vi "Write System State Ref.vi"(8 "error in (no error)":errorcluster, 10 "System Status Ref":refnum<vi>, 11 "System Actor in":refnum<class "System Actor.lvclass">) -> (0 "error out":errorcluster, 3 "System Actor out":refnum<class "System Actor.lvclass">)   [LabVIEW 2014, in "Robot Actor Framework.lvlib" / "System Actor.lvlib" / "System Actor.lvclass"]
uses:
  System Actor.lvclass
  System State.ctl
  Command Actor/Command Actor Class/Command State.ctl
  Command Actor/Command Actor Class/Command States.ctl
  Command Processor Actor/Command Processor Actor Class/Command Processor State.ctl
  Command Processor Actor/Command Processor Actor Class/Command Processor States.ctl
  System Actor.lvclass/System Actor.ctl
  Command Actor/Command Actor Class/Command Actor.lvclass
  Command Processor Actor/Command Processor Actor Class/Command Processor Actor.lvclass
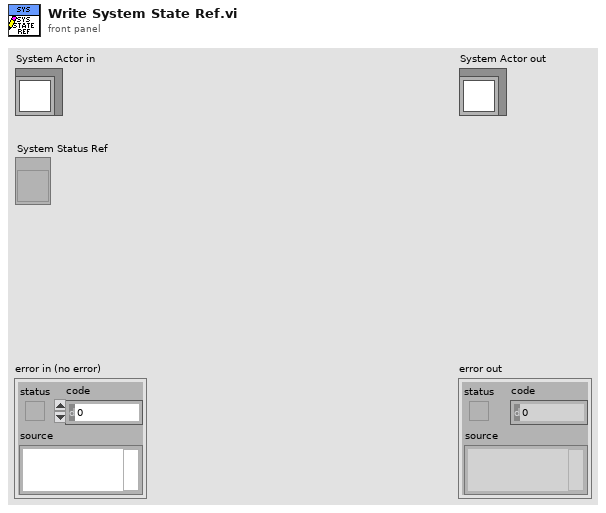
[diagram p1: front panel]
types:
  T1 = typedef "Robot Actor Framework.lvlib/System Actor.lvlib/System Actor.lvclass/System State.ctl" = cluster{"Instance Name":string, "Current Command Status":T2, "System Start Time":timestamp, "Next Command ID":dbl, "Command Processor Status":T4}
  T2 = typedef "Robot Actor Framework.lvlib/Command Actor.lvlib/Command Actor.lvclass/Command State.ctl" = cluster{"Command Name":string, "Command Start Time":timestamp, "Command End Time":timestamp, "Is Command Finished?":bool, "Command ID":u32, "Command State":T3, "Command State Time":timestamp}
  T3 = typedef "Robot Actor Framework.lvlib/Command Actor.lvlib/Command Actor.lvclass/Command States.ctl" = enum16{"Unknown", "Started", "Stopped", "Finished"}
  T4 = typedef "Robot Actor Framework.lvlib/Command Processor Actor.lvlib/Command Processor Actor.lvclass/Command Processor State.ctl" = cluster{"Current State":T5, "Last State Update":timestamp, "Queued Commands":u32, "Current Command Status":T2, "Previous State":T5, "Current State Entry":timestamp, "Transitioning State":bool, "Commands Behind":dbl, "Last Command Queue Time":timestamp}
  T5 = typedef "Robot Actor Framework.lvlib/Command Processor Actor.lvlib/Command Processor Actor.lvclass/Command Processor States.ctl" = enum16{"Unknown", "No Command", "Running Command", "Starting Command", "Stopping Command", "Finishing Command"}
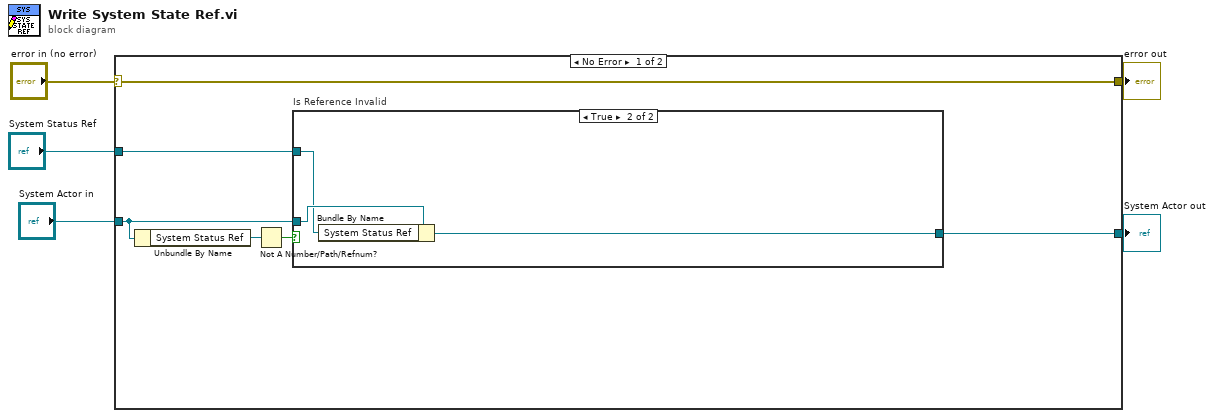
[diagram p0: block diagram]
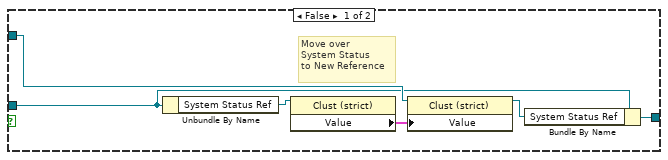
[diagram p2: hidden frame]
diagram:
  n1 = case shown="No Error" "error in (no error)" {
    selector: "error in (no error)" -> [w11 w21]
    tunnel: [w11 w21] -> w4
    tunnel: [w10 w22] -> w2
    tunnel: "System Actor in" -> [w8 w22]
    tunnel: "System Status Ref" -> [w9 _]
    frame No Error {
      n2 = Unbundle By Name(w8) -> ("System Status Ref"=w7:refnum<vi>)
      n3 = Not A Number/Path/Refnum?(number/path/refnum=w7) -> (NaN/Path/Refnum?=w6:bool)
      n4 = case "Is Reference Invalid" shown="True" w6 {
        tunnel: w8 -> [w14 w20]
        tunnel: [w13 w19] -> w10
        tunnel: w9 -> [w16 w18]
        frame False {
          # "Move over\nSystem Status\nto New Reference"
          n5 = Unbundle By Name(w14) -> ("System Status Ref"=w17:refnum<vi>)
          n6 = property class="Clust (strict)"(reference=w17) -> ("Value"=w15:T1)  [unwired: 1 in, 2 out]
          n7 = property class="Clust (strict)"(reference=w16, "Value"=w15) -> (reference out=w12:refnum<vi>)  [unwired: 1 in, 1 out]
          n8 = Bundle By Name(cluster=w14, "System Status Ref"=w12) -> (w13:refnum<class "System Actor.lvclass">)
        }
        frame True {
          n9 = Bundle By Name(cluster=w20, "System Status Ref"=w18) -> (w19:refnum<class "System Actor.lvclass">)
        }
      }
    }
    frame Error {
    }
  }
  "error out" <- w4
  "System Actor out" <- w2
